vi "GetTurbidity.vi"(1 "DMM (to sample) GPIB address:":string="11", 3 "Sample Temperature Controller GPIB address:":string="15", 6 "File path:":path=path "c:/Data", 7 "Tmax (K):":dbl=50.0 format="%.3f", 9 "Tmin (K):":dbl=35.0 format="%.3f", 10 "Sample name (date):":string="MCS_CritOpal_063016d", 13 "Allowable temperature deviation (K):":dbl=0.005 format="%.4f", 17 "Measurement wait time (ms):":dbl=150.0, 19 "Number of voltage measurements\nbetween temperature check:":dbl=10.0) -> (11 "Number of isotherms (>1):":dbl=128.00000000000003)   [LabVIEW 2014]
panel:
  in  "Voltage Resolution (mV)":dbl=1.0 format="%.2f"
  in  "Delta T":dbl=0.1 format="%.3f"
  in  "DMM2 GPIB address:":string="22"
  # "Make sure the temperature controller has been correctly setup before running this VI"
  # "(c) 2001 Thomas Frederiksen"
  # "Get Turbidity"
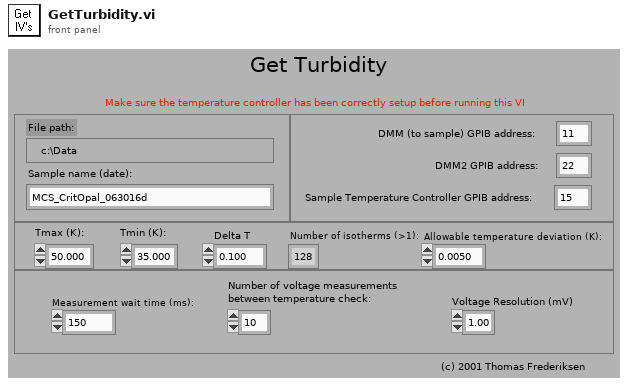
[diagram p1: front panel]
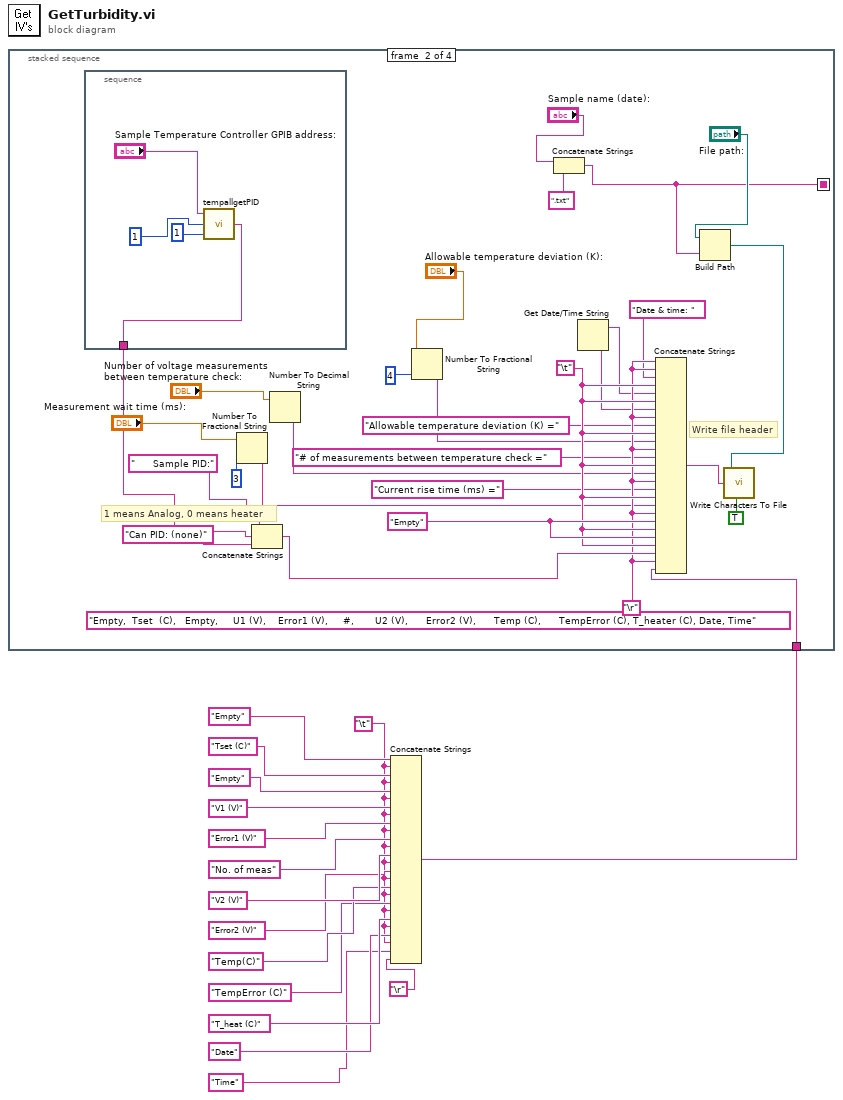
[diagram p0: block diagram]
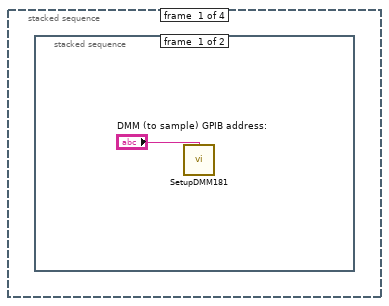
[diagram p2: hidden frame]
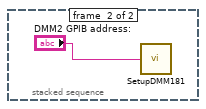
[diagram p3: hidden frame]
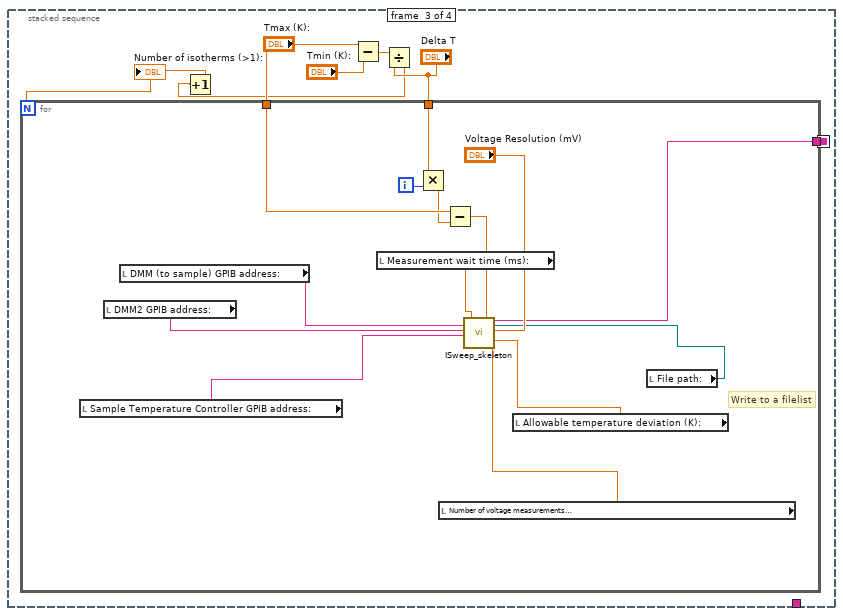
[diagram p4: hidden frame]
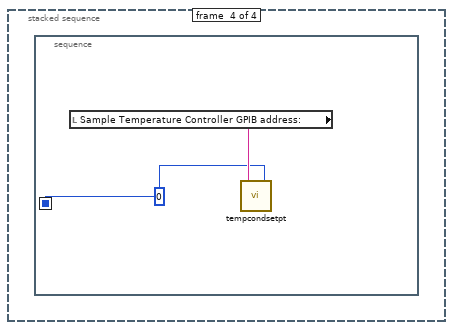
[diagram p5: hidden frame]
diagram:
  w4 = "\t"
  n1 = Concatenate Strings("Empty", w4, "Tset (C)", w4, "Empty", w4, "V1 (V)", w4, "Error1 (V)", w4, "No. of meas", w4, "V2 (V)", w4, "Error2 (V)", w4, "Temp(C)", w4, "TempError (C)", w4, "T_heat (C)", w4, "Date", w4, "Time", "\r") -> (w1:string)
  n2 = stacked-sequence {
    seq-local: [_ w24 _ _] -> [_ _ w52 _]
    tunnel: w1 -> [_ w19 _ _]
    frame #0 {
      n3 = stacked-sequence {
        frame #0 {
          n4 = call "SetupDMM181.vi"("DMM GPIB Address"="DMM (to sample) GPIB address:") -> ()
        }
        frame #1 {
          n5 = call "SetupDMM181.vi"("DMM GPIB Address"="DMM2 GPIB address:") -> ()
        }
      }
    }
    frame #1 {
      w47 = "Empty"
      w45 = "\t"
      (unwired) "Empty,  Tset  (C),   Empty,     U1 (V),    Error1 (V),     #,       U2 (V),      Error2 (V),      Temp (C),      TempError (C), T_heater (C), Date, Time"
      w41 = "\r"
      # "1 means Analog, 0 means heater"
      # "Write file header"
      n6 = stacked-sequence {
        tunnel: [w49] -> w46
        frame #0 {
          n7 = call "tempallgetPID.vi"("Neocera: Heater or Analog;\nLakeshore: Heater 1 or 2"=1, "Temperature controller"=1, "GPIB address"="Sample Temperature Controller GPIB address:") -> ("Out"=w49:string)
        }
      }
      n8 = Number To Fractional String(number="Measurement wait time (ms):", precision (6)=3) -> (F-format string=w39:string)  [unwired: 2 in]
      n9 = Concatenate Strings("      Sample PID:", w46, "Can PID: (none)") -> (w44:string)
      n10 = Number To Decimal String(number="Number of voltage measurements\nbetween temperature check:") -> (decimal integer string=w33:string)  [unwired: 1 in]
      n11 = Number To Fractional String(number="Allowable temperature deviation (K):", precision (6)=4) -> (F-format string=w31:string)  [unwired: 2 in]
      n12 = Concatenate Strings("Sample name (date):", ".txt") -> (w24:string)
      n13 = Get Date/Time String() -> (date string=w36:string, time string=w37:string)  [unwired: 3 in]
      n14 = Concatenate Strings(w41, w41, "Date & time: ", w45, w36, w45, w37, w41, "Allowable temperature deviation (K) =", w45, w31, w41, "# of measurements between temperature check =", w45, w33, w41, "Current rise time (ms) =", w45, w39, w41, w47, w45, w47, w45, w44, w41, w19) -> (w29:string)
      n15 = Build Path(base path="File path:", name or relative path=w24) -> (appended path=w23:path)
      n16 = call <vilib>:"Write Characters To File.vi"("append to file? (new file:F)"=TRUE, "character string"=w29, "file path (dialog if empty)"=w23) -> ()  [unwired: 2 in, 1 out]
    }
    frame #2 {
      n17 = Subtract(x="Tmax (K):", y="Tmin (K):") -> (x-y=w58:dbl)
      n18 = Divide(x=w58, y="Delta T") -> (x/y=w54:dbl)
      n19 = Increment(x=w54) -> (x+1=w53:dbl)
      "Number of isotherms (>1):" <- w53
      n20 = for {
        N: w53 -> [_]
        tunnel: "Delta T" -> [w71]
        tunnel: "Tmax (K):" -> [w70]
        tunnel: w52 -> [w63]
        i -> [w72]
        # "Write to a filelist"
        n21 = local read "Sample Temperature Controller GPIB address:"() -> (w59:string)
        n22 = local read "DMM2 GPIB address:"() -> (w67:string)
        n23 = local read "DMM (to sample) GPIB address:"() -> (w66:string)
        n24 = local read "Measurement wait time (ms):"() -> (w60:dbl)
        n25 = Multiply(x=w71, y=w72) -> (x*y=w69:dbl)
        n26 = local read "Number of voltage measurements\nbetween temperature check:"() -> (w62:dbl)
        n27 = Subtract(x=w70, y=w69) -> (x-y=w68:dbl)
        n28 = local read "Allowable temperature deviation (K):"() -> (w61:dbl)
        n29 = local read "File path:"() -> (w64:path)
        n30 = call "ISweep_skeleton.vi"("DMM1 GPIB address"=w66, "DMM2 GPIB address"=w67, "Main Temperature Controller GPIB address"=w59, "Measurement wai time (ms)"=w60, "Setpoint temperature (K)"=w68, "File Name"=w63, "File Path"=w64, "Voltage resolution (mV)"="Voltage Resolution (mV)", "Allowable temperature deviation (K)"=w61, "Number of voltage measurements\nbetween temperature check"=w62) -> ()  [unwired: 10 in]
      }
    }
    frame #3 {
      n31 = stacked-sequence {
        seq-local: [w73] -> [_]
        frame #0 {
          w73 = 0
          n32 = local read "Sample Temperature Controller GPIB address:"() -> (w74:string)
          n33 = call "tempcondsetpt.vi"("Set Point"=w73, "GPIB Address"=w74) -> ()  [unwired: 1 in, 1 out]
        }
      }
    }
  }
